vi "Initialize Server State.vi"(8 "error in":errorcluster, 10 "Initial State":T1, 11 "gRPC Server in":refnum<class "Servicer.lvclass">) -> (0 "error out":errorcluster, 3 "gRPC Server out":refnum<class "Servicer.lvclass">)   [LabVIEW 2019, in "gRPC-servicer.lvlib" / "Servicer.lvclass"]
uses:
  Servicer.lvclass
  Server State Data.ctl
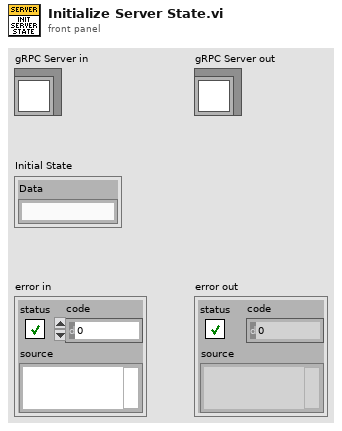
[diagram p1: front panel]
types:
  T1 = typedef "gRPC-servicer.lvlib/Servicer.lvclass/Server State Data.ctl" = cluster{"Data":string}
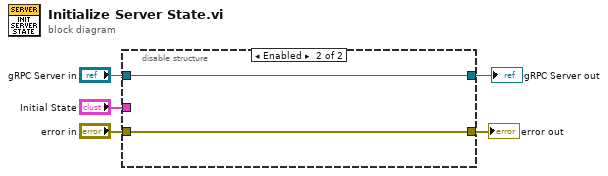
[diagram p0: block diagram]
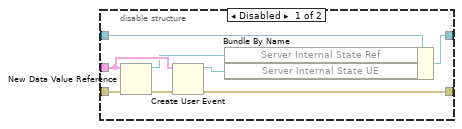
[diagram p2: hidden frame]
diagram:
  n1 = disable-structure shown="Enabled" {
    disable-tunnel: "error in" -> [w13 w15]
    disable-tunnel: [w12 w15] -> w4
    disable-tunnel: "gRPC Server in" -> [w11 w14]
    disable-tunnel: [w10 w14] -> w2
    disable-tunnel: "Initial State" -> [w9 _]
    frame Disabled {
      n2 = New Data Value Reference(data value=w9, error in=w13) -> (data value reference=w6:refnum<data-value>, error out=w8:errorcluster)
      n3 = Create User Event(user event datatype=w9, error in=w8) -> (user event=w7:refnum<user-event>, error out=w12:errorcluster)
      n4 = Bundle By Name(cluster=w11, "Server Internal State Ref"=w6, "Server Internal State UE"=w7) -> (w10:refnum<class "Servicer.lvclass">)
    }
    frame Enabled {
    }
  }
  "error out" <- w4
  "gRPC Server out" <- w2
